vi "Read Document Source.vi"(8 "error in (no error)":errorcluster, 11 "WebView2 Control in":refnum<class "WebView2 Control.lvclass">) -> (0 "error out":errorcluster, 2 "DocumentSource":string, 3 "WebView2 Control out":refnum<class "WebView2 Control.lvclass">)   [LabVIEW 2020, in "WebView2.lvlib" / "WebView2 Control.lvclass"]
uses:
  WebView2 Control.lvclass
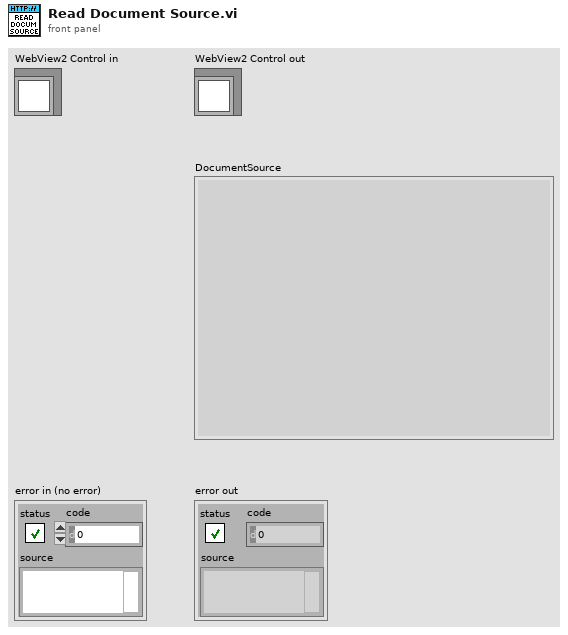
[diagram p1: front panel]
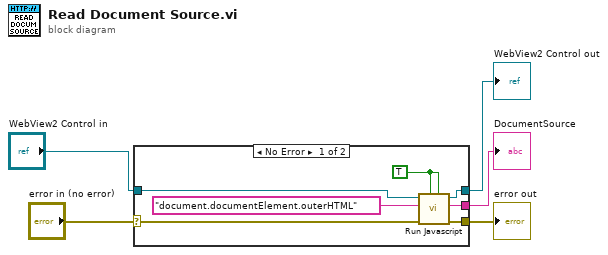
[diagram p0: block diagram]
diagram:
  n1 = case shown="No Error" "error in (no error)" {
    selector: "error in (no error)" -> [w12 w14]
    tunnel: [w11 w14] -> w4
    tunnel: [w9 w13] -> w2
    tunnel: "WebView2 Control in" -> [w10 w13]
    tunnel: [w6 _] -> w1
    frame No Error {
      w7 = TRUE ("Fetch Result (T)")
      n2 = call "Run Javascript.vi"("Decode Result (T)"=w7, "Fetch Result (T)"=w7, "error in (no error)"=w12, "javaScript"="document.documentElement.outerHTML", "WebView2 Control in"=w10) -> ("error out"=w11:errorcluster, "Result"=w6:string, "WebView2 Control out"=w9:refnum<class "WebView2 Control.lvclass">)  [unwired: 4 in]
    }
    frame Error {
    }
  }
  "error out" <- w4
  "WebView2 Control out" <- w2
  "DocumentSource" <- w1
